vi "subDFD_Generate QAM Signal.vi"(6 "delay":i32=1, 9 "order":i32=39, 10 "#band":i32=4, 11 "#signal":i32=512) -> (2 "transmitted signal":cdb[][](array[numeric]), 3 "delayed transmitted signal":cdb[][](array[numeric]))   [LabVIEW 2023]
uses:
  <vilib>/addons/Digital Filter Design/Process.llb/DFD Integer Delay (Array NChan).vi
  <vilib>/ptbypt/NI_PtbyPt.lvlib
  <vilib>/addons/Digital Filter Design/NI_DigFilterLicensed.lvlib
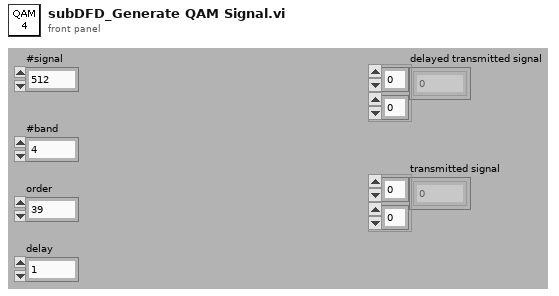
[diagram p1: front panel]
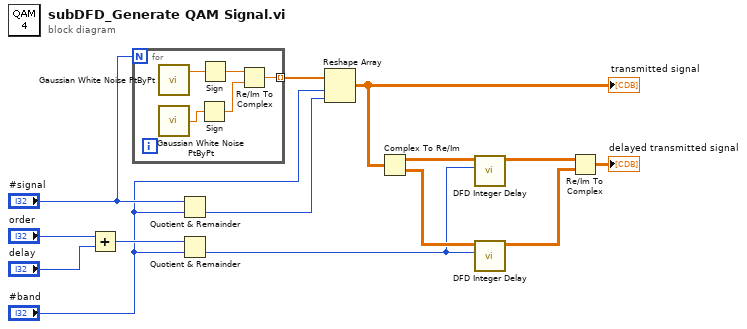
[diagram p0: block diagram]
diagram:
  n1 = Add(x="order", y="delay") -> (x+y=w7:i32)
  n2 = for {
    N: "#signal" -> [_]
    tunnel: [w15] -> w12 mode=indexing
    n3 = call <vilib>:"Gaussian White Noise PtByPt.vi"() -> ("Gaussian white noise"=w17:dbl)  [unwired: 3 in]
    n4 = call <vilib>:"Gaussian White Noise PtByPt.vi"() -> ("Gaussian white noise"=w19:dbl)  [unwired: 3 in]
    n5 = Sign(1:w19) -> (0:w18:dbl)
    n6 = Sign(1:w17) -> (0:w16:dbl)
    n7 = Re/Im To Complex(1:w18, 2:w16) -> (0:w15:cdb)
  }
  n8 = Quotient & Remainder(x="#signal", y="#band") -> (floor(x/y)=w13:i32)  [unwired: 1 out]
  n9 = Quotient & Remainder(x=w7, y="#band") -> (floor(x/y)=w4:i32)  [unwired: 1 out]
  n10 = Reshape Array(w12, "#band", w13) -> (w11:cdb[][])
  "transmitted signal" <- w11
  n11 = Complex To Re/Im(x + iy=w11) -> (x=w10:dbl[][], y=w5:dbl[][])
  n12 = call-poly <vilib>:"DFD Integer Delay.vi"("delay"=w4, "signal in"=w10) -> ("signal out"=w3:dbl[][])  [unwired: 8 in, 1 out]
  n13 = call-poly <vilib>:"DFD Integer Delay.vi"("delay"=w4, "signal in"=w5) -> ("signal out"=w2:dbl[][])  [unwired: 8 in, 1 out]
  n14 = Re/Im To Complex(1:w2, 2:w3) -> (0:→"delayed transmitted signal":cdb[][])
